vi "Create Channel Buffer.vi"(8 "error in":errorcluster, 10 "Channel":string, 11 "Buffer Lossless Dig in":refnum<class "Buffer Lossless Digital.lvclass">) -> (0 "error out":errorcluster, 3 "Buffer Lossless Dig out":refnum<class "Buffer Lossless Digital.lvclass">)   [LabVIEW 2024, in "Buffer Lossless Digital.lvclass"]
uses:
  Buffer Lossless Digital.lvclass
  Buffer Lossless Digital.lvclass/Buffer Lossless Digital.ctl
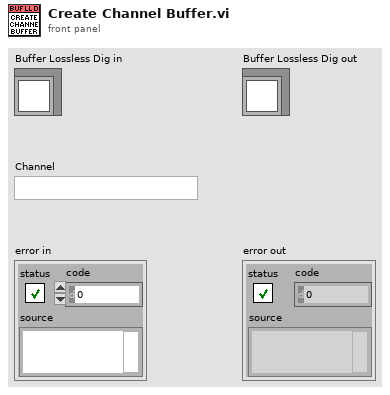
[diagram p1: front panel]
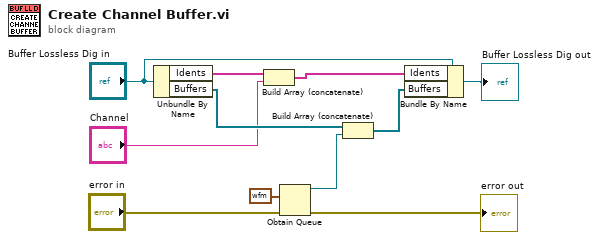
[diagram p0: block diagram]
diagram:
  n1 = Unbundle By Name("Buffer Lossless Dig in") -> ("Idents"=w10:string[], "Buffers"=w11:refnum<queue>[])
  n2 = Build Array (concatenate)(w10, "Channel") -> (w9:string[])
  n3 = Obtain Queue(element data type=digitalwaveform {"t0"=timestamp(0 s since 1904-01-01), "dt"=1.0, "Y"={"transitions"=[], "data"=[]}} ("output waveform"), error in (no error)="error in") -> (queue out=w1:refnum<queue>, error out=→"error out":errorcluster)  [unwired: 3 in, 1 out]
  n4 = Build Array (concatenate)(w11, w1) -> (w8:refnum<queue>[])
  n5 = Bundle By Name(cluster="Buffer Lossless Dig in", "Idents"=w9, "Buffers"=w8) -> (→"Buffer Lossless Dig out":refnum<class "Buffer Lossless Digital.lvclass">)
